vi "ATS_Search_Spec.vi"(8 "Rate / Range":bool, 9 "Treshold (30)":u32=30, 10 "Value In":u32, 11 "StringArray":string[](array[string])=["1 kS/s", "2 kS/s", "5 kS/s", "10 kS/s", "20 kS/s", "50 kS/s", "100 kS/s", "200 kS/s", "500 kS/s", "1 MS/s", "2 MS/s", "5 MS/s", "10 MS/s", "20 MS/s", "25 MS/s", "50 MS/s", "100 MS/s", "200 MS/s", "500 MS/s", "1 GS/s"]) -> (0 "Result":u32, 1 "Index":u32, 2 "Out_Value":u32, 3 "String":string, 4 ">Treshold":bool)   [LabVIEW 2015]
doc: "_____AlazarTech, Scope_____\n\nSearch, in the StringArray the ValueIn.\nIf the Value input is Higher than treshold than search the closest value\nIf not search the Index \"Value_In\" limited by the Maximum index in the StringArray input.\n\nResult is of same \"type\" as the ValueIn, Index if lower than Treshold or Out_Value otherwise."
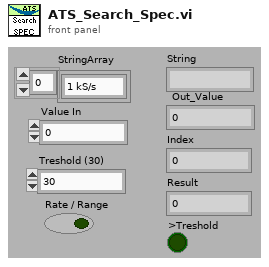
[diagram p1: front panel]
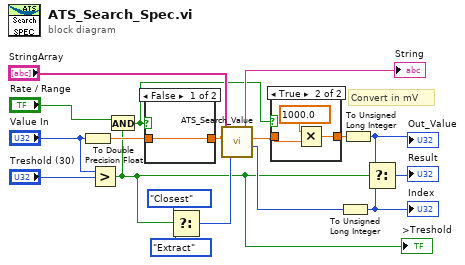
[diagram p0: block diagram]
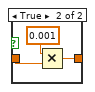
[diagram p3: hidden frame]
diagram:
  # "Convert in mV"
  n1 = To Double Precision Float(number="Value In") -> (double precision float=w6:dbl)
  n2 = Greater?(x="Value In", y="Treshold (30)") -> (0:w4:bool)
  ">Treshold" <- w4
  n3 = And(x="Rate / Range", y=w4) -> (x .and. y?=w1:bool)
  n4 = case shown="False" w1 {
    tunnel: w6 -> [w19 w21]
    tunnel: [w19 w22] -> w5
    frame False {
    }
    frame True {
      n5 = Multiply(x=0.001, y=w21) -> (x*y=w22:dbl)
    }
  }
  n6 = Select(t=enum16{"Extract", "Equal", "Closest"}."Closest" ("Search_Mode"), s=w4, f=enum16{"Extract", "Equal", "Closest"}."Extract" ("Search_Mode")) -> (s? t:f=w14:enum16{"Extract", "Equal", "Closest"})
  n7 = call "ATS_Search_Value.vi"("Search_Mode"=w14, "Value In"=w5, "StringArray"="StringArray") -> ("Index"=w10:i32, "Out_Value"=w3:dbl, "String"=→"String":string)  [unwired: 2 in]
  n8 = case shown="True" w1 {
    tunnel: w3 -> [w23 w25]
    tunnel: [w23 w26] -> w2
    frame False {
    }
    frame True {
      n9 = Multiply(x=1000.0, y=w25) -> (x*y=w26:dbl)
    }
  }
  n10 = To Unsigned Long Integer(number=w10) -> (unsigned 32bit integer=w8:u32)
  "Index" <- w8
  n11 = To Unsigned Long Integer(number=w2) -> (unsigned 32bit integer=w11:u32)
  "Out_Value" <- w11
  n12 = Select(t=w11, s=w4, f=w8) -> (s? t:f=→"Result":u32)
